vi "delta z to index.vi"(7 "number of points":i32, 10 "complex region":T1, 11 "z":cdb) -> (2 "im index":i32, 3 "re index":i32)   [LabVIEW 2010]
uses:
  complex region.ctl
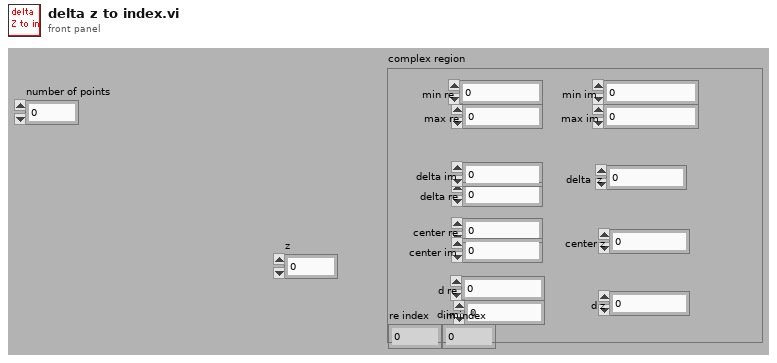
[diagram p1: front panel]
types:
  T1 = typedef "complex region.ctl" = cluster{"max re":dbl, "min re":dbl, "max im":dbl, "min im":dbl, "delta re":dbl, "delta im":dbl, "center re":dbl, "delta  z":cdb, "center im":dbl, "center z":cdb, "d im":dbl, "d re":dbl, "d z":cdb}
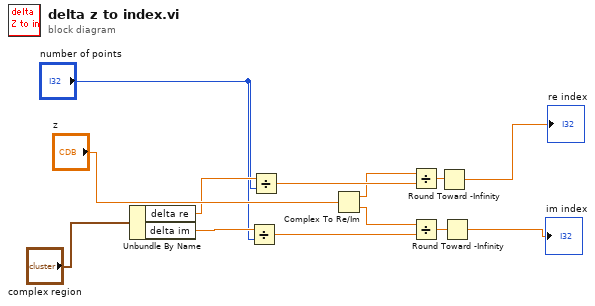
[diagram p0: block diagram]
diagram:
  n1 = Unbundle By Name("complex region") -> ("delta re"=w7:dbl, "delta im"=w5:dbl)
  n2 = Divide(x=w5, y="number of points") -> (x/y=w3:dbl)
  n3 = Divide(x=w7, y="number of points") -> (x/y=w6:dbl)
  n4 = Complex To Re/Im(x + iy="z") -> (x=w2:dbl, y=w1:dbl)
  n5 = Divide(x=w2, y=w6) -> (x/y=w13:dbl)
  n6 = Divide(x=w1, y=w3) -> (x/y=w12:dbl)
  n7 = Round Toward -Infinity(1:w13) -> (0:→"re index":dbl)
  n8 = Round Toward -Infinity(1:w12) -> (0:→"im index":dbl)
